vi "Read Connection Lookup.vi"(8 "error in (no error)":errorcluster, 11 "Abstract Routing Channel Template in":refnum<class "Abstract Routing Channel Template.lvclass">) -> (0 "error out":errorcluster, 2 "Routing Templates.lvlib:Abstract Connection Lookup.lvclass":refnum<class "Abstract Connection Lookup.lvclass">, 3 "Abstract Routing Channel Template out":refnum<class "Abstract Routing Channel Template.lvclass">)   [LabVIEW 2020, in "Routing Templates.lvlib" / "Abstract Routing Channel Template.lvclass"]
uses:
  Abstract Routing Channel Template.lvclass
  Abstract Routing Channel Template.lvclass/Abstract Routing Channel Template.ctl
  Connection Lookups/Abstract Connection Lookup/Abstract Connection Lookup.lvclass
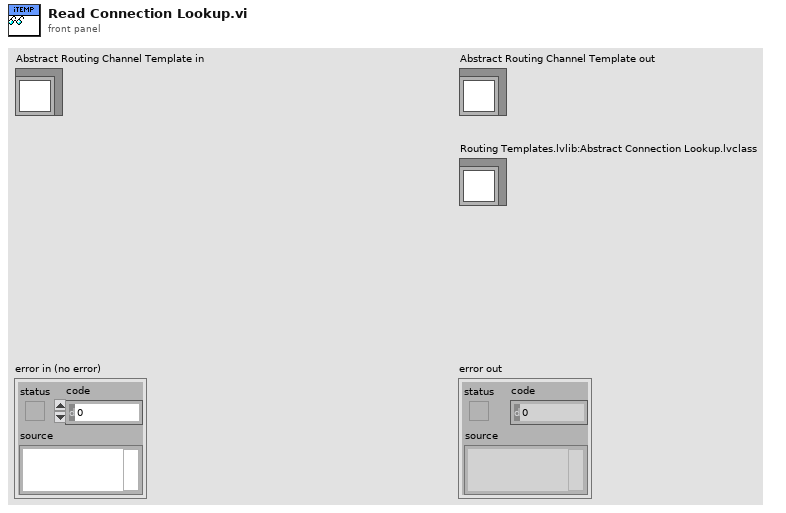
[diagram p1: front panel]
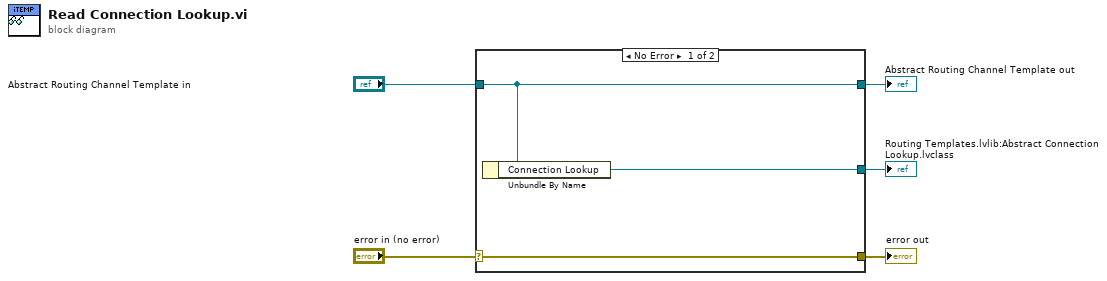
[diagram p0: block diagram]
diagram:
  n1 = case shown="No Error" "error in (no error)" {
    selector: "error in (no error)" -> [w8 w9]
    tunnel: [w8 w9] -> w4
    tunnel: [w7 w10] -> w2
    tunnel: "Abstract Routing Channel Template in" -> [w7 w10]
    tunnel: [w6 _] -> w1
    frame No Error {
      n2 = Unbundle By Name(w7) -> ("Connection Lookup"=w6:refnum<class "Abstract Connection Lookup.lvclass">)
    }
    frame Error {
    }
  }
  "error out" <- w4
  "Abstract Routing Channel Template out" <- w2
  "Routing Templates.lvlib:Abstract Connection Lookup.lvclass" <- w1
